vi "LiveAcquisition.vi"() -> ()   [LabVIEW 2020]
uses:
  C:/Users/Hannah/Documents/GitHub/pan-ASLM/LabVIEW camera PVCam/Dependencies/PVCamNET.dll
  Dependencies/PVCamNET.dll
panel:
  out "Captured Frames":i64
  in  "?":bool
  in  "?":bool
  in  "Exposure time":u32=5
  # "LiveAcqusition.vi\n\nDescription:\nThis sample code lets the user use live mode \nwith the user's preferred exposure time.\n\nSteps to run:\n1. Click \"Run\"\n2. Enter exposure time\n3. Click \"START\"\n4. Click \"STOP\""
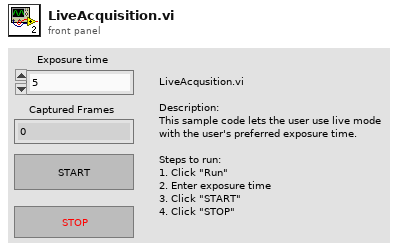
[diagram p1: front panel]
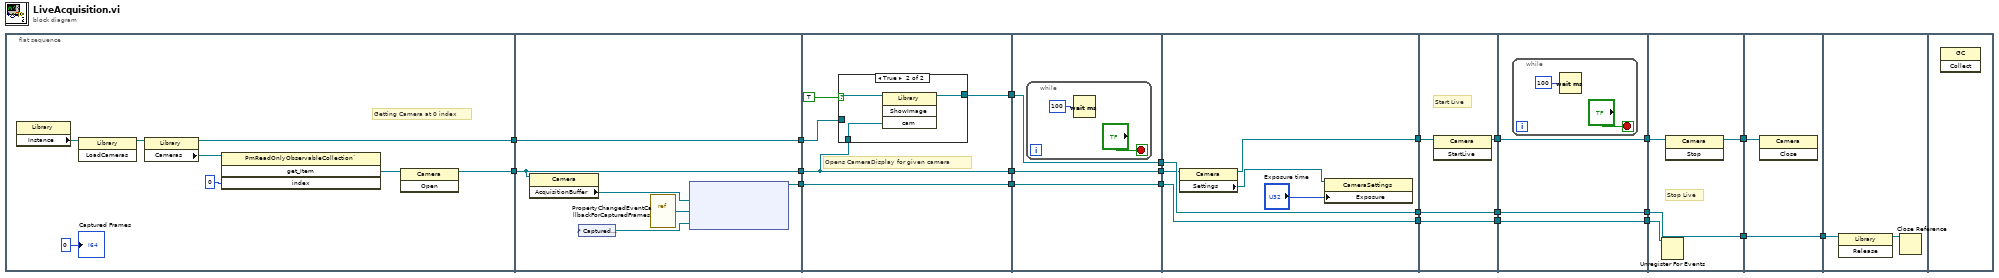
[diagram p0: block diagram]
diagram:
  n1 = flat-sequence {
    tunnel: [w27] -> w11
    tunnel: [w28] -> w9
    tunnel: w11 -> [w37]
    tunnel: [w37] -> w10
    tunnel: w9 -> [w36]
    tunnel: [w36] -> w8
    tunnel: [w32] -> w2
    tunnel: w10 -> [w42]
    tunnel: w8 -> [w38]
    tunnel: [w38] -> w15
    tunnel: [w41] -> w13
    tunnel: [w40] -> w3
    tunnel: w2 -> [w40]
    tunnel: w15 -> [w49]
    tunnel: [w49] -> w14
    tunnel: w13 -> [w48]
    tunnel: [w48] -> w12
    tunnel: [w47] -> w4
    tunnel: w3 -> [w47]
    tunnel: [w57] -> w17
    tunnel: w12 -> [w57]
    tunnel: w14 -> [w56]
    tunnel: [w53] -> w5
    tunnel: w4 -> [w53]
    tunnel: [w52] -> w1
    tunnel: [w60] -> w23
    tunnel: [w59] -> w18
    tunnel: w17 -> [w59]
    tunnel: [w58] -> w6
    tunnel: w5 -> [w58]
    tunnel: w1 -> [w61]
    tunnel: w23 -> [w64]
    tunnel: [w64] -> w22
    tunnel: [w63] -> w19
    tunnel: w18 -> [w63]
    tunnel: [w62] -> w7
    tunnel: w6 -> [w62]
    tunnel: w22 -> [w70]
    tunnel: [w69] -> w21
    tunnel: [w68] -> w20
    tunnel: w19 -> [w68]
    tunnel: w7 -> [w67]
    tunnel: w21 -> [w72]
    tunnel: w20 -> [w71]
    tunnel: [w71] -> w16
    tunnel: w16 -> [w74]
    frame #0 {
      # "Getting Camera at 0 index"
      n2 = property class="Library"() -> ("Instance"=w25:refnum<k24>)  [unwired: 2 in, 2 out]
      n3 = invoke class="Library" method="LoadCameras"(reference=w25) -> (reference out=w24:refnum<k24>)  [unwired: 2 in, 2 out]
      n4 = property class="Library"(reference=w24) -> (reference out=w27:refnum<k24>, "Cameras"=w31:refnum<k24>)  [unwired: 1 in, 1 out]
      n5 = invoke class="PmReadOnlyObservableCollection`" method="get_Item"(reference=w31, "index"=0) -> ("get_Item"=w29:refnum<k24>)  [unwired: 2 in, 3 out]
      n6 = invoke class="Camera" method="Open"(reference=w29) -> (reference out=w28:refnum<k24>)  [unwired: 2 in, 2 out]
      "Captured Frames" <- i64 0 ("Captured (Library counter)")
    }
    frame #1 {
      n7 = property class="Camera"(reference=w36) -> ("AcquisitionBuffer"=w35:refnum<k24>)  [unwired: 1 in, 2 out]
      n8 = control-ref of="Captured Frames"() -> (w34:refnum<vi>)
      n9 = vi-ref "PropertyChangedEventCallbackForCapturedFrames.vi"() -> ("vi reference"=w33:refnum<vi>)
      n10 = node(w35, w33, w34) -> (w32:refnum<k27>)  [unwired: 2 in, 1 out]
    }
    frame #2 {
      # "Opens CameraDisplay for given camera"
      n11 = case shown="True" TRUE {
        tunnel: w42 -> [w43 w46]
        tunnel: [w43 w45] -> w41
        tunnel: w38 -> [_ w44]
        frame False {
        }
        frame True {
          n12 = invoke class="Library" method="ShowImage"(reference=w46, "cam"=w44) -> (reference out=w45:refnum<k24>)  [unwired: 2 in, 3 out]
        }
      }
    }
    frame #3 {
      n13 = while {
        stop <- "?" stop-if-true
        n14 = Wait (ms)(milliseconds to wait=u32 100) -> ()  [unwired: 1 out]
      }
    }
    frame #4 {
      n15 = property class="Camera"(reference=w56) -> (reference out=w52:refnum<k24>, "Settings"=w54:refnum<k24>)  [unwired: 1 in, 1 out]
      n16 = property class="CameraSettings"(reference=w54, "Exposure"="Exposure time") -> ()  [unwired: 1 in, 2 out]
    }
    frame #5 {
      # "Start Live"
      n17 = invoke class="Camera" method="StartLive"(reference=w61) -> (reference out=w60:refnum<k24>)  [unwired: 2 in, 2 out]
    }
    frame #6 {
      n18 = while {
        stop <- "?" stop-if-true
        n19 = Wait (ms)(milliseconds to wait=u32 100) -> ()  [unwired: 1 out]
      }
    }
    frame #7 {
      # "Stop Live"
      n20 = Unregister For Events(event registration refnum=w67) -> ()  [unwired: 1 in, 1 out]
      n21 = invoke class="Camera" method="Stop"(reference=w70) -> (reference out=w69:refnum<k24>)  [unwired: 2 in, 2 out]
    }
    frame #8 {
      n22 = invoke class="Camera" method="Close"(reference=w72) -> ()  [unwired: 2 in, 3 out]
    }
    frame #9 {
      n23 = invoke class="Library" method="Release"(reference=w74) -> (reference out=w73:refnum<k24>)  [unwired: 2 in, 2 out]
      n24 = Close Reference(reference=w73) -> ()  [unwired: 1 in, 1 out]
    }
    frame #10 {
      n25 = invoke class="GC" method="Collect"() -> ()  [unwired: 3 in, 3 out]
    }
  }
